vi "GetSubjectUI.vi"(0 "Enable":bool=TRUE, 5 "error in (no error)":errorcluster) -> (14 "subjectSelected":string, 18 "OK":bool, 19 "error out":errorcluster)   [LabVIEW 2014]
doc: "Displays a standard dialog box that prompts users to enter information, such as a user name and password.\n--------------------\n\nThis Express VI is configured as follows:\n\nMessage to Display to the User:\nThe inputs are: \nCheckbox: Andy\nCheckbox: Apollo\nCheckbox: Ben\nCheckbox: Charles\nCheckbox: Claude\nCheckbox: Leo\nCheckbox: Woody"
panel:
  in  "Mouse":bool caption="Woody"
  in  "Woody":bool
  in  "Leo":bool
  in  "Claude":bool
  in  "Charles":bool
  in  "Ben":bool
  in  "Apollo":bool
  in  "Andy":bool
  out "String":string
  in  "Cancel":bool
  in  "OK2":bool
  in  "OK1":bool
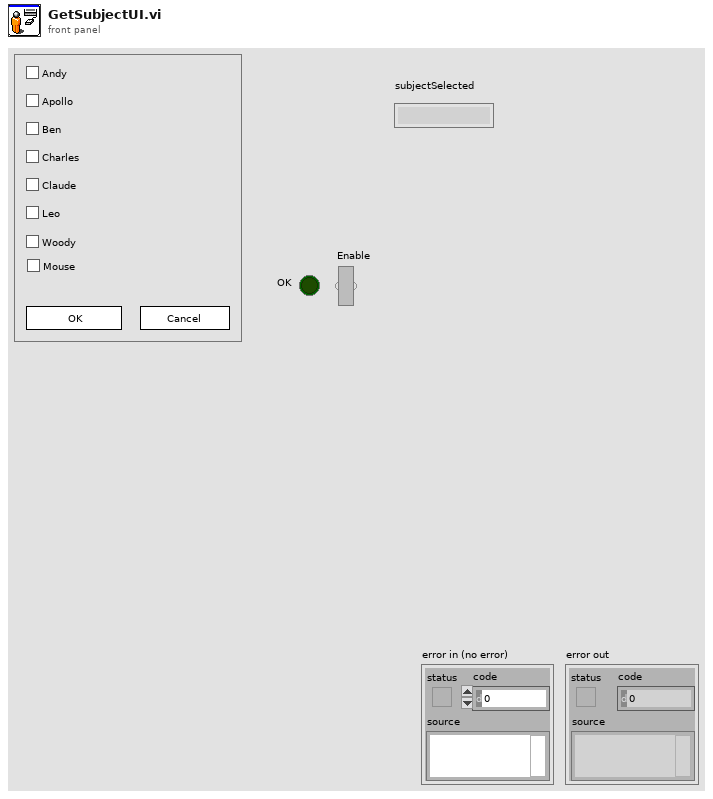
[diagram p1: front panel]
types:
  T1 = cluster{"Input Name":string, "Input Data Type":i32}[]
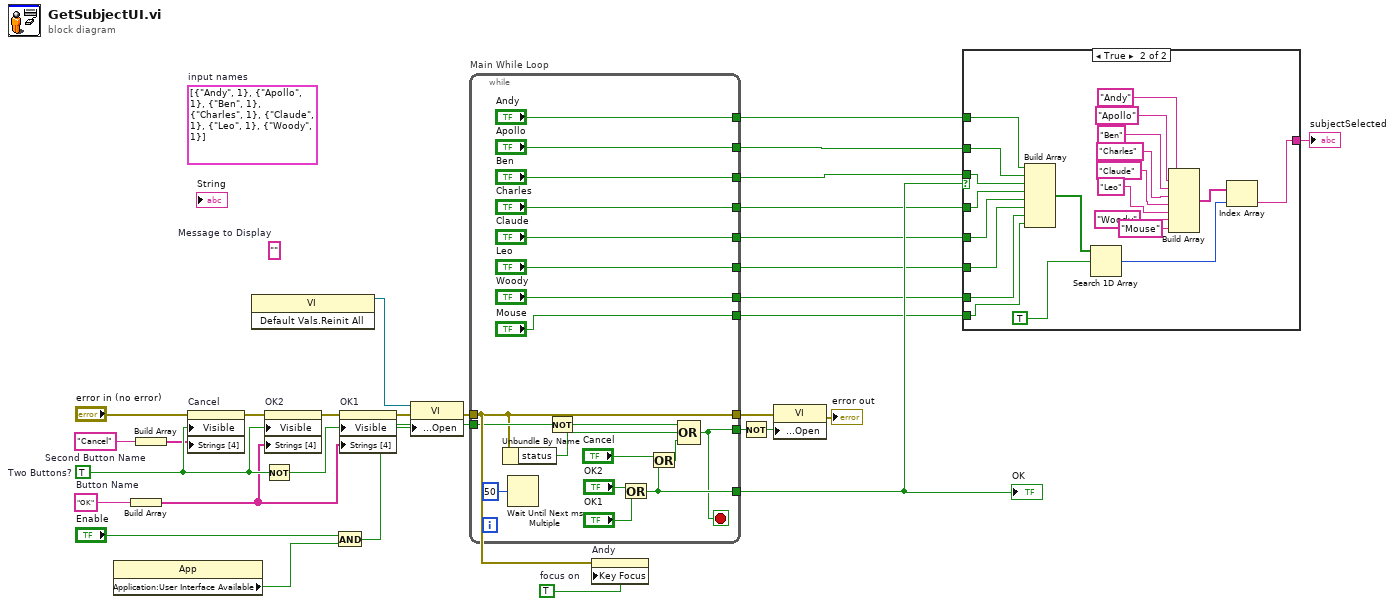
[diagram p0: block diagram]
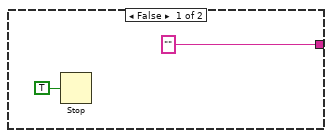
[diagram p2: hidden frame]
diagram:
  w11 = TRUE  # focus on
  (unwired) T1 [{"Input Name"="Andy", "Input Data Type"=1}, {"Input Name"="Apollo", "Input Data Type"=1}, {"Input Name"="Ben", "Input Data Type"=1}, {"Input Name"="Charles", "Input Data Type"=1}, {"Input Name"="Claude", "Input Data Type"=1}, {"Input Name"="Leo", "Input Data Type"=1}, {"Input Name"="Woody", "Input Data Type"=1}]  # input names
  w23 = "Cancel"  # Second Button Name
  w21 = "OK"  # Button Name
  (unwired) ""  # Message to Display
  w30 = TRUE  # Two Buttons?
  n1 = property class="App"() -> ("Application:User Interface Available"=w13:bool)  [unwired: 2 in, 2 out]
  n2 = Build Array(w21) -> (w22:string[])
  n3 = Build Array(w23) -> (w24:string[])
  n4 = property on="Cancel" class="Bool"(error in="error in (no error)", "Visible"=w30, "Strings [4]"=w24) -> (error out=w28:errorcluster)  [unwired: 1 in, 1 out]
  n5 = invoke class="VI" method="Default Vals.Reinit All"() -> (reference out=w12:refnum<vi>)  [unwired: 3 in, 2 out]
  n6 = Not(x=w30) -> (.not. x?=w29:bool)
  n7 = property on="OK2" class="Bool"(error in=w28, "Visible"=w30, "Strings [4]"=w22) -> (error out=w27:errorcluster)  [unwired: 1 in, 1 out]
  n8 = And(x="Enable", y=w13) -> (x .and. y?=w14:bool)
  n9 = property on="OK1" class="Bool"(error in=w27, "Visible"=w29, "Strings [4]"=w22) -> (error out=w20:errorcluster)  [unwired: 1 in, 1 out]
  n10 = property class="VI"(reference=w12, error in=w20, "Front Panel Window:Open"=w14) -> (error out=w19:errorcluster)  [unwired: 1 out]
  n11 = while "Main While Loop" {
    tunnel: [w46] -> w9
    tunnel: w14 -> [w44]
    tunnel: [w42] -> w25
    tunnel: w19 -> [w41]
    tunnel: [w41] -> w17
    tunnel: ["Andy"] -> w10
    tunnel: ["Apollo"] -> w8
    tunnel: ["Ben"] -> w7
    tunnel: ["Charles"] -> w6
    tunnel: ["Claude"] -> w5
    tunnel: ["Leo"] -> w4
    tunnel: ["Woody"] -> w3
    tunnel: ["Mouse"] -> w1
    stop <- w42 stop-if-true
    n12 = Unbundle By Name(w41) -> ("status"=w39:bool)
    n13 = Wait Until Next ms Multiple(millisecond multiple=u32 50) -> ()  [unwired: 1 out]
    n14 = Not(x=w44) -> (.not. x?=w43:bool)
    n15 = Or(x="OK2", y="OK1") -> (x .or. y?=w46:bool)
    n16 = Or(x="Cancel", y=w46) -> (x .or. y?=w40:bool)
    n17 = Compound Arithmetic op=OR(w43, w39, w40) -> (w42:bool)
  }
  "OK" <- w9
  n18 = property on="Andy" class="Bool (strict)"(error in=w19, "Key Focus"=w11) -> ()  [unwired: 1 in, 2 out]
  n19 = Not(x=w25) -> (.not. x?=w26:bool)
  n20 = property class="VI"(error in=w17, "Front Panel Window:Open"=w26) -> (error out=→"error out":errorcluster)  [unwired: 1 in, 1 out]
  n21 = case shown="True" w9 {
    tunnel: ["" w64] -> w2
    tunnel: w10 -> [_ w61]
    tunnel: w8 -> [_ w60]
    tunnel: w7 -> [_ w59]
    tunnel: w6 -> [_ w58]
    tunnel: w5 -> [_ w57]
    tunnel: w4 -> [_ w56]
    tunnel: w3 -> [_ w55]
    tunnel: w1 -> [_ w53]
    frame False {
      n22 = Stop(stop? (T)=TRUE) -> ()
    }
    frame True {
      n23 = Build Array(w61, w60, w59, w58, w57, w56, w55, w53) -> (w63:bool[])
      n24 = Search 1D Array(1D array=w63, element=TRUE) -> (index of element=w62:i32)  [unwired: 1 in]
      n25 = Build Array("Andy", "Apollo", "Ben", "Charles", "Claude", "Leo", "Woody", "Mouse" ("element")) -> (w72:string[])
      n26 = Index Array(array=w72, index=w62) -> (element=w64:string)
    }
  }
  "subjectSelected" <- w2
